vi "M05 Hydraulics.vi"(11 "NXT/EV3":T1) -> (3 "NXT/EV3":T1)   [LabVIEW 2016]
uses:
  <vilib>/NXT/Subs/LVHSConnector.ctl
  <vilib>/NXT/LegoClasses/BrickReference/BrickReference.lvclass
  <vilib>/NXT/Block Support/NXT_InputPort.ctl
  <vilib>/NXT/Dual Mode Library/Waits/Wait_Num.vi
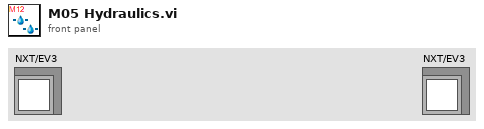
[diagram p1: front panel]
types:
  T1 = typedef "LVHSConnector.ctl" = refnum<class "BrickReference.lvclass">
  T2 = typedef "NXT_InputPort.ctl" = u32
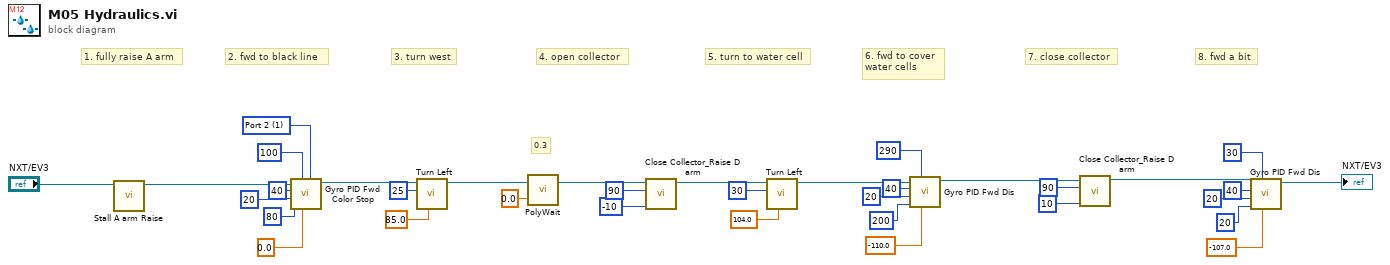
[diagram p0: block diagram]
diagram:
  w25 = T2 1 items=["Port 1", "Port 2", "Port 3", "Port 4"] ("Port")
  # "8. fwd a bit"
  # "7. close collector"
  # "6. fwd to cover\nwater cells"
  # "5. turn to water cell"
  # "0.3"
  # "4. open collector"
  # "3. turn west"
  # "2. fwd to black line"
  # "1. fully raise A arm"
  n1 = call "Stall A arm Raise.vi"("NXT/EV3"="NXT/EV3") -> ("NXT/EV3"=w26:T1)  [unwired: 10 in]
  n2 = call "Gyro PID Fwd Color Stop.vi"("Port"=w25, "Target angle"=sgl 0.0, "Threshold to Color"=100, "Threshold to slow"=80, "Min. speed"=20, "Max. speed"=40, "EV3 in"=w26) -> ("EV3 out"=w19:T1)  [unwired: 4 in]
  n3 = call "Turn Left.vi"("Turning angle"=sgl 85.0, "Motor B (right)"=i8 25, "EV3 in"=w19) -> ("EV3 out"=w18:T1)  [unwired: 8 in]
  n4 = call-poly <vilib>:"PolyWait.vi"("Time (1 sec)"=sgl 0.0, "NXT/EV3"=w18) -> ("NXT/EV3"=w6:T1)  [unwired: 2 in]
  n5 = call "Close Collector_Raise D arm.vi"("Power"=i8 -10 ("Speed 1"), "Rotation"=90 ("Distance 1"), "EV3 in"=w6) -> ("EV3 out"=w5:T1)  [unwired: 8 in]
  n6 = call "Turn Left.vi"("Turning angle"=sgl 104.0, "Motor B (right)"=i8 30, "EV3 in"=w5) -> ("EV3 out"=w15:T1)  [unwired: 8 in]
  n7 = call "Gyro PID Fwd Dis.vi"("Target angle"=sgl -110.0, "Threshold to stop"=290, "Threshold to slow"=200, "Min. speed"=20, "Max. speed"=40, "EV3 in"=w15) -> ("EV3 out"=w3:T1)  [unwired: 5 in]
  n8 = call "Close Collector_Raise D arm.vi"("Power"=i8 10 ("Speed 1"), "Rotation"=90 ("Distance 1"), "EV3 in"=w3) -> ("EV3 out"=w1:T1)  [unwired: 8 in]
  n9 = call "Gyro PID Fwd Dis.vi"("Target angle"=sgl -107.0, "Threshold to stop"=30, "Threshold to slow"=20, "Min. speed"=20, "Max. speed"=40, "EV3 in"=w1) -> ("EV3 out"=→"NXT/EV3":T1)  [unwired: 5 in]
